vi "screen for job logs.vi"() -> ()   [LabVIEW 2022 SP3]
panel:
  out "Duration":timestamp format="%<%Hh:%Mm:%Ss>T"
  out "Job name":string
  in  "return":bool
  out "total cycles":dbl
  out "total steps":dbl
  out "total procedures":dbl
  out "Total jobs":dbl
  out "Ended on":timestamp format="%<%d/%m/%y | %H:%M>T"
  out "started on":timestamp format="%<%d/%m/%y | %H:%M>T"
  out "user name":string
  out "1D Array":timestamp[](array[timestamp]) format="%<%d/%m/%y | %H:%M>T"
  out "Data array":dbl[][](array[numeric])
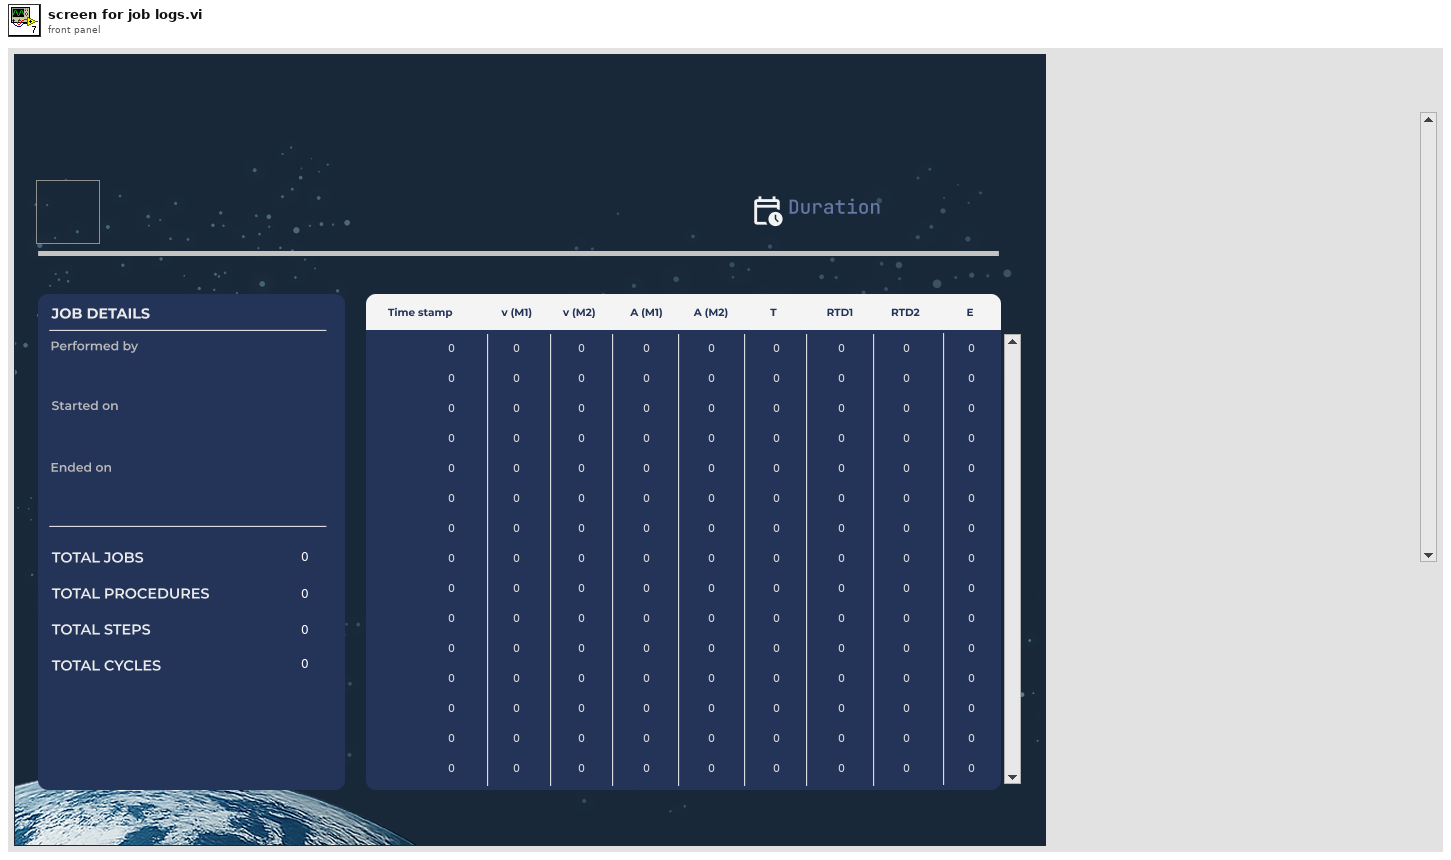
[diagram p1: front panel]
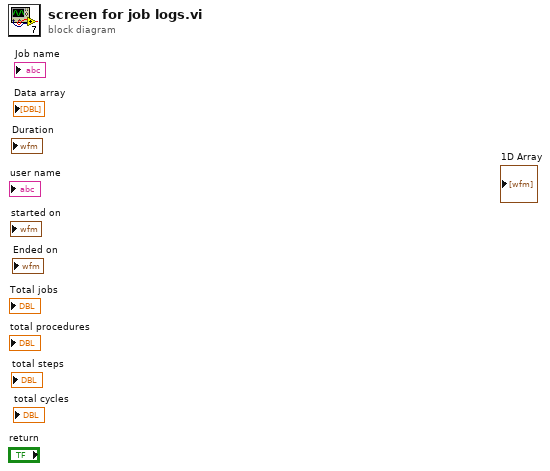
[diagram p0: block diagram]
diagram:
